vi "Checkers Board Setup.vi"() -> (3 "new picture":picture)   [LabVIEW 2014]
uses:
  <vilib>/Utility/miscctls.llb/LVPositionTypeDef.ctl
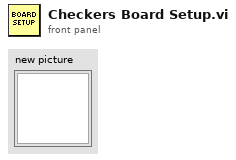
[diagram p1: front panel]
types:
  T1 = typedef "LVPositionTypeDef.ctl" = cluster{"Left":i32, "Top":i32}
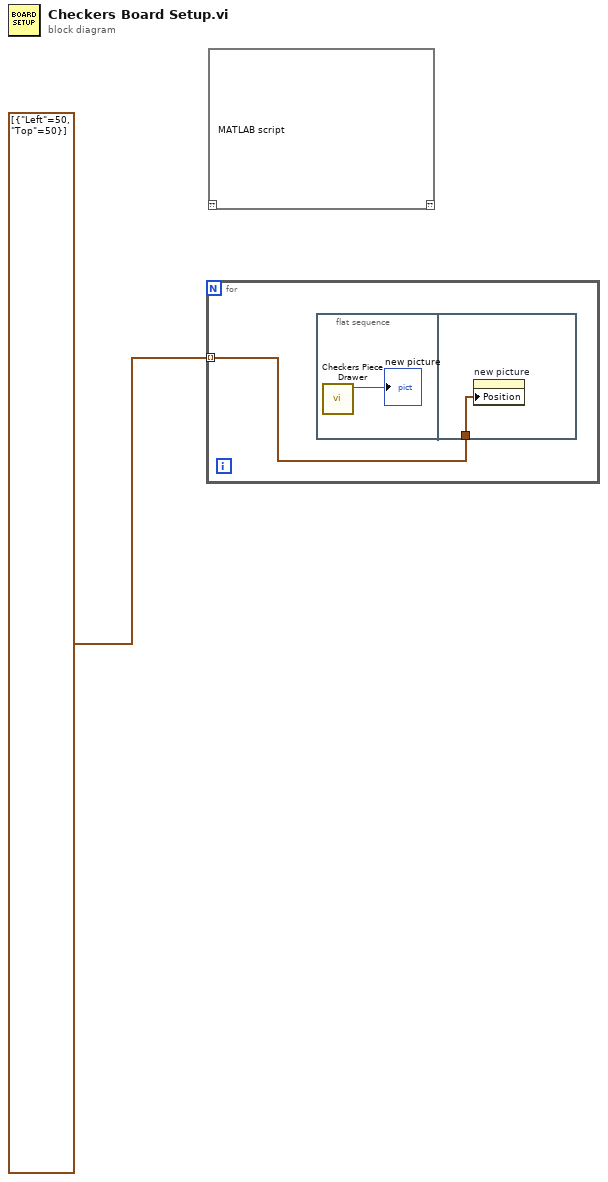
[diagram p0: block diagram]
diagram:
  n1 = for {
    tunnel: T1[] [{"Left"=50, "Top"=50}] -> [w2] mode=indexing
    n2 = flat-sequence {
      tunnel: w2 -> [w4]
      frame #0 {
        n3 = call "Checkers Piece Drawer.vi"() -> ("new picture"=→"new picture":picture)  [unwired: 11 in]
      }
      frame #1 {
        n4 = property on="new picture" class="Pict"("Position"=w4) -> ()  [unwired: 2 in, 2 out]
      }
    }
  }
  n5 = script code="MATLAB script"() -> ()  [unwired: 1 in, 1 out]
